vi "IIC Init.vi"(9 "pConfig":T1, 10 "IICIndex":i32, 11 "DevHandle":i32) -> (1 "pConfig out":T1, 3 "function return":i32)   [LabVIEW 2010, in "usb2iic.lvlib"]
doc: "int WINAPI IIC_Init(int DevHandle,int IICIndex, PIIC_CONFIG pConfig);"
uses:
  usb2iic.lvlib
  USB2XXX.dll
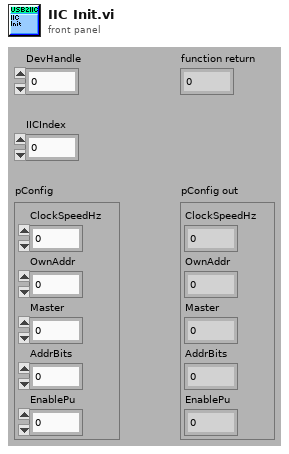
[diagram p1: front panel]
types:
  T1 = cluster{"ClockSpeedHz":u32, "OwnAddr":u16, "Master":u8, "AddrBits":u8, "EnablePu":u8}
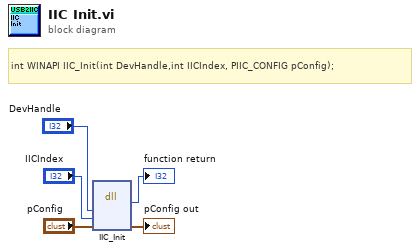
[diagram p0: block diagram]
diagram:
  # "int WINAPI IIC_Init(int DevHandle,int IICIndex, PIIC_CONFIG pConfig);"
  n1 = dll-call lib="G:/OtherWork/USB2XXX_Example/trunk/Labview/PublicFiles/usb2iic/USB2XXX.*" fn="IIC_Init"("DevHandle"="DevHandle", "IICIndex"="IICIndex", "pConfig"="pConfig") -> (→"function return":i32, "pConfig"=→"pConfig out":T1)  [unwired: 5 in, 2 out]
